vi "Limit String Demo.vi"() -> ()   [LabVIEW 2013]
uses:
  Limit String.xctl
panel:
  in  "Limit String":string(xcontrol)
  out "字符串":string
  in  "停止":bool
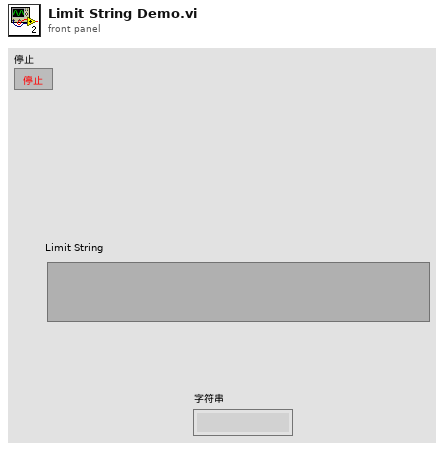
[diagram p1: front panel]
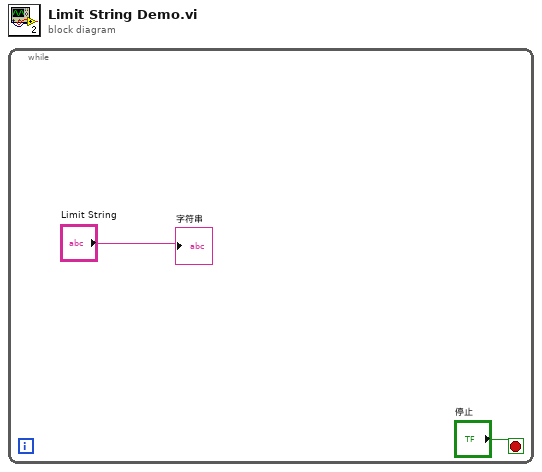
[diagram p0: block diagram]
diagram:
  n1 = while {
    stop <- "停止" stop-if-true
    "字符串" <- "Limit String"
  }
